vi "close modules.vi"(11 "close FP?":bool) -> ()   [LabVIEW 2012]
panel:
  out "Array":errorcluster[](array[cluster])
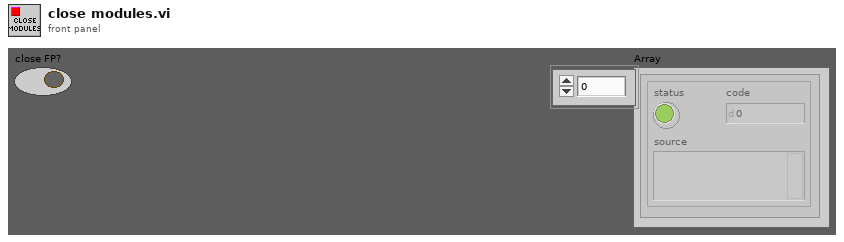
[diagram p1: front panel]
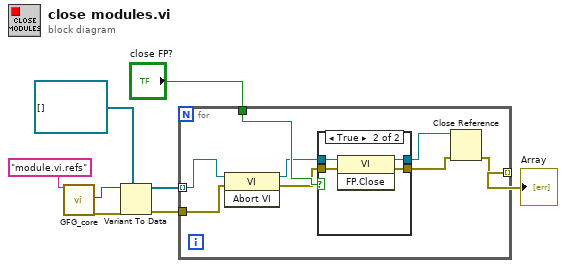
[diagram p0: block diagram]
diagram:
  n1 = call "GFG_core.vi"("Variable Name in"="module.vi.refs") -> ("Variant Out"=w6:variant, "error out"=w7:errorcluster)  [unwired: 12 in, 5 out]
  n2 = Variant To Data(error in=w7, type=refnum<vi>[] [], Variant=w6) -> (data=w4:refnum<vi>[], error out=w3:errorcluster)
  n3 = for {
    tunnel: w4 -> [w15] mode=indexing
    tunnel: w3 -> [w12]
    tunnel: [w9] -> w2 mode=indexing
    tunnel: "close FP?" -> [w16]
    n4 = invoke class="VI" method="Abort VI"(reference=w15, error in=w12) -> (reference out=w14:refnum<vi>, error out=w13:errorcluster)  [unwired: 1 in, 1 out]
    n5 = case shown="True" w16 {
      tunnel: w14 -> [w18 w22]
      tunnel: [w18 w21] -> w11
      tunnel: [w17 w20] -> w10
      tunnel: w13 -> [w17 w19]
      frame False {
      }
      frame True {
        n6 = invoke class="VI" method="FP.Close"(reference=w22, error in=w19) -> (reference out=w21:refnum<vi>, error out=w20:errorcluster)  [unwired: 1 in, 1 out]
      }
    }
    n7 = Close Reference(reference=w11, error in (no error)=w10) -> (error out=w9:errorcluster)
  }
  "Array" <- w2
